vi "CRYUnits Conversion.vi"(7 "Axis to change units":enum16{"x", "y", "z"}(ring), 8 "New dB ref":dbl=1.0 format="%.1f", 9 "Custom unit in":string, 10 "New data (dB/Lin)":u16(ring)=1 items=["dB", "Lin"], 11 "Data in":T1={"Name"="", "Curve"=[], "X data"=1, "Y data"=1, "Z data"=1, "X axis"=0, "Y axis"=1, "Z axis"=1, "X unit"="Hz", "Y unit"="", "Z unit"="deg.", "X dB ref"=1.0, "Y dB ref"=1.0, "Z dB ref"=1.0, "single val"=FALSE, "protected"=FALSE, "display X"=TRUE, "display Y"=TRUE, "display Z"=TRUE, "Test Info"="", "Step No."=0, "Plot Settings"={"Color"=0, "Interpolation"=0, "Point Style"=0, "Line Style"=0, "Point Color"=0, "Line Width"=0, "Bar Plot Style"=0, "Fill To"=0}, "AutoProtect"=FALSE} {"Z data" items=["dB", "Lin"]; "X data" items=["dB", "Lin"]; "Y data" items=["dB", "Lin"]; "Z dB ref" format="%.1f"; "Z axis" items=["Log", "Lin"]; "X dB ref" format="%.1f"; "X axis" items=["Log", "Lin"]; "Y axis" items=["Log", "Lin"]; "Y dB ref" format="%.1f"; "Curve"."z" format="%.2f"; "Curve"."y" format="%.2f"; "Curve"."x" format="%.2f"}) -> (3 "Data with new units":T1={"Name"="", "Curve"=[], "X data"=1, "Y data"=1, "Z data"=1, "X axis"=0, "Y axis"=1, "Z axis"=1, "X unit"="Hz", "Y unit"="", "Z unit"="deg.", "X dB ref"=1.0, "Y dB ref"=1.0, "Z dB ref"=1.0, "single val"=FALSE, "protected"=FALSE, "display X"=TRUE, "display Y"=TRUE, "display Z"=TRUE, "Test Info"="", "Step No."=0, "Plot Settings"={"Color"=0, "Interpolation"=0, "Point Style"=0, "Line Style"=0, "Point Color"=0, "Line Width"=0, "Bar Plot Style"=0, "Fill To"=0}, "AutoProtect"=FALSE} {"Z data" items=["dB", "Lin"]; "X data" items=["dB", "Lin"]; "Y data" items=["dB", "Lin"]; "Z dB ref" format="%.1f"; "Z axis" items=["Log", "Lin"]; "X dB ref" format="%.1f"; "X axis" items=["Log", "Lin"]; "Y axis" items=["Log", "Lin"]; "Y dB ref" format="%.1f"; "Curve"."z" format="%.2f"; "Curve"."y" format="%.2f"; "Curve"."x" format="%.2f"})   [LabVIEW 2013]
uses:
  Typedef Control/CRYData Cluster.ctl
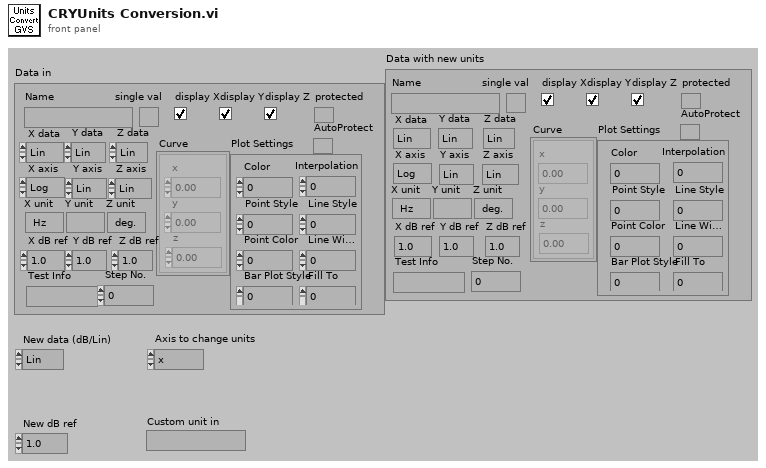
[diagram p1: front panel]
types:
  T1 = typedef "CRYData Cluster.ctl" = cluster{"Name":string, "Curve":cluster{"x":dbl, "y":dbl, "z":dbl}[], "X data":u16, "Y data":u16, "Z data":u16, "X axis":u16, "Y axis":u16, "Z axis":u16, "X unit":string, "Y unit":string, "Z unit":string, "X dB ref":dbl, "Y dB ref":dbl, "Z dB ref":dbl, "single val":bool, "protected":bool, "display X":bool, "display Y":bool, "display Z":bool, "Test Info":string, "Step No.":i32, "Plot Settings":cluster{"Color":u32, "Interpolation":u8, "Point Style":u8, "Line Style":u8, "Point Color":u32, "Line Width":u8, "Bar Plot Style":u8, "Fill To":i16}, "AutoProtect":bool}
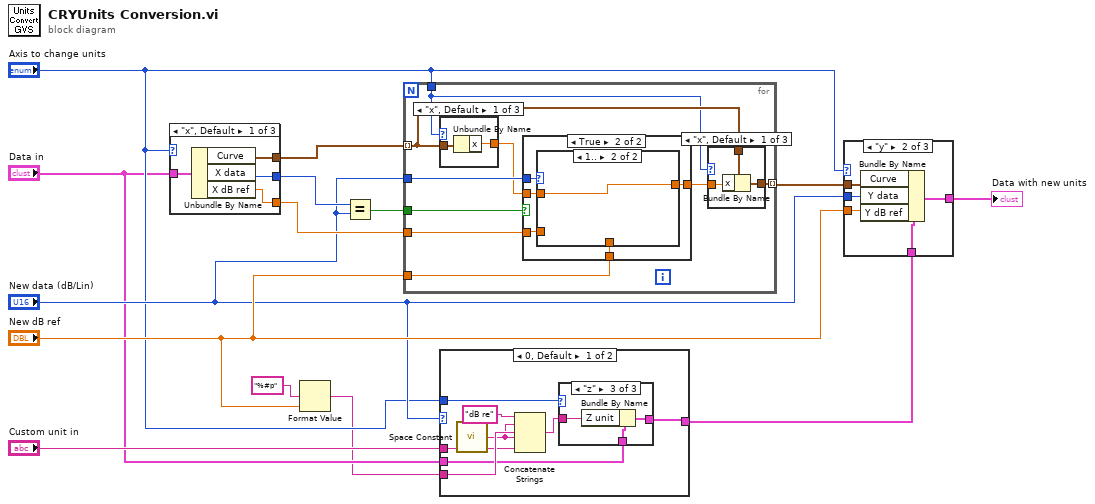
[diagram p0: block diagram]
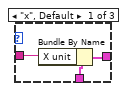
[diagram p2: hidden frame]
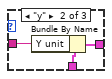
[diagram p3: hidden frame]
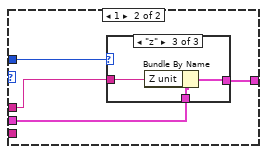
[diagram p4: hidden frame]
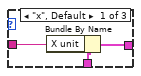
[diagram p5: hidden frame]
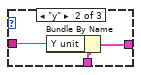
[diagram p6: hidden frame]
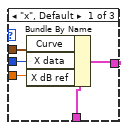
[diagram p7: hidden frame]
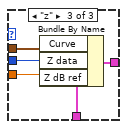
[diagram p8: hidden frame]
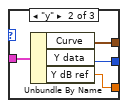
[diagram p9: hidden frame]
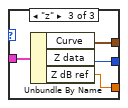
[diagram p10: hidden frame]
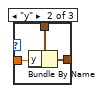
[diagram p11: hidden frame]
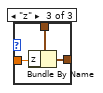
[diagram p12: hidden frame]
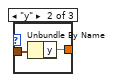
[diagram p13: hidden frame]
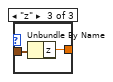
[diagram p14: hidden frame]
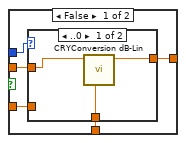
[diagram p15: hidden frame]
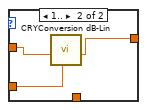
[diagram p16: hidden frame]
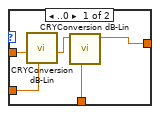
[diagram p17: hidden frame]
diagram:
  n1 = case shown="\"x\", Default" "Axis to change units" {
    tunnel: [w18 w22 w26] -> w12
    tunnel: [w17 w21 w25] -> w10
    tunnel: "Data in" -> [w16 w20 w24]
    tunnel: [w15 w19 w23] -> w11
    frame "x", Default {
      n2 = Unbundle By Name(w16) -> ("Curve"=w15:cluster{"x":dbl, "y":dbl, "z":dbl}[], "X data"=w17:u16, "X dB ref"=w18:dbl)
    }
    frame "y" {
      n3 = Unbundle By Name(w20) -> ("Curve"=w19:cluster{"x":dbl, "y":dbl, "z":dbl}[], "Y data"=w21:u16, "Y dB ref"=w22:dbl)
    }
    frame "z" {
      n4 = Unbundle By Name(w24) -> ("Curve"=w23:cluster{"x":dbl, "y":dbl, "z":dbl}[], "Z data"=w25:u16, "Z dB ref"=w26:dbl)
    }
  }
  n5 = Format Value(format string="%#p", value (0)="New dB ref") -> (output string=w2:string)  [unwired: 1 out]
  n6 = Equal?(x=w10, y="New data (dB/Lin)") -> (x = y?=w14:bool)
  n7 = for {
    tunnel: w14 -> [w35]
    tunnel: w11 -> [w32] mode=indexing
    tunnel: "New dB ref" -> [w29]
    tunnel: w12 -> [w34]
    tunnel: "New data (dB/Lin)" -> [w33]
    tunnel: [w30] -> w13 mode=indexing
    tunnel: "Axis to change units" -> [w27]
    n8 = case shown="\"x\", Default" w27 {
      tunnel: w32 -> [w46 w48 w50]
      tunnel: [w45 w47 w49] -> w28
      frame "x", Default {
        n9 = Unbundle By Name(w46) -> ("x"=w45:dbl)
      }
      frame "y" {
        n10 = Unbundle By Name(w48) -> ("y"=w47:dbl)
      }
      frame "z" {
        n11 = Unbundle By Name(w50) -> ("z"=w49:dbl)
      }
    }
    n12 = case shown="True" w35 {
      tunnel: [w55 w66] -> w31
      tunnel: w28 -> [w54 w65]
      tunnel: w29 -> [w53 w63]
      tunnel: w34 -> [w52 w62]
      tunnel: w33 -> [w51 w64]
      frame False {
        n13 = case shown="..0" w51 {
          tunnel: w53 -> [w58 _]
          tunnel: w54 -> [w56 w60]
          tunnel: [w57 w59] -> w55
          tunnel: w52 -> [_ w61]
          frame ..0 {
            n14 = call "CRYConversion dB-Lin.vi"("dB ref."=w58, "Lin In"=w56) -> ("Log Out"=w57:dbl)  [unwired: 4 in, 3 out]
          }
          frame 1.. {
            n15 = call "CRYConversion dB-Lin.vi"("dB ref."=w61, "Log In"=w60) -> ("Lin Out"=w59:dbl)  [unwired: 4 in, 3 out]
          }
        }
      }
      frame True {
        n16 = case shown="1.." w64 {
          tunnel: w65 -> [w71 w72]
          tunnel: [w69 w72] -> w66
          tunnel: w63 -> [w68 _]
          tunnel: w62 -> [w70 _]
          frame ..0 {
            n17 = call "CRYConversion dB-Lin.vi"("dB ref."=w70, "Log In"=w71) -> ("Lin Out"=w67:dbl)  [unwired: 4 in, 3 out]
            n18 = call "CRYConversion dB-Lin.vi"("dB ref."=w68, "Lin In"=w67) -> ("Log Out"=w69:dbl)  [unwired: 4 in, 3 out]
          }
          frame 1.. {
          }
        }
      }
    }
    n19 = case shown="\"x\", Default" w27 {
      tunnel: w32 -> [w38 w41 w44]
      tunnel: w31 -> [w37 w40 w43]
      tunnel: [w36 w39 w42] -> w30
      frame "x", Default {
        n20 = Bundle By Name(cluster=w38, "x"=w37) -> (w36:cluster{"x":dbl, "y":dbl, "z":dbl})
      }
      frame "y" {
        n21 = Bundle By Name(cluster=w41, "y"=w40) -> (w39:cluster{"x":dbl, "y":dbl, "z":dbl})
      }
      frame "z" {
        n22 = Bundle By Name(cluster=w44, "z"=w43) -> (w42:cluster{"x":dbl, "y":dbl, "z":dbl})
      }
    }
  }
  n23 = case shown="0, Default" "New data (dB/Lin)" {
    tunnel: "Custom unit in" -> [w75 w93]
    tunnel: [w79 w92] -> w1
    tunnel: w2 -> [w77 _]
    tunnel: "Data in" -> [w74 w91]
    tunnel: "Axis to change units" -> [w73 w90]
    frame 0, Default {
      n24 = call <vilib>:"Space Constant.vi"() -> ("String"=w76:string)
      n25 = Concatenate Strings("dB re" ("string"), w76, w77, w76, w75) -> (w80:string)
      n26 = case shown="\"z\"" w73 {
        tunnel: w80 -> [w83 w86 w89]
        tunnel: [w81 w85 w87] -> w79
        tunnel: w74 -> [w82 w84 w88]
        frame "x", Default {
          n27 = Bundle By Name(cluster=w82, "X unit"=w83) -> (w81:T1)
        }
        frame "y" {
          n28 = Bundle By Name(cluster=w84, "Y unit"=w86) -> (w85:T1)
        }
        frame "z" {
          n29 = Bundle By Name(cluster=w88, "Z unit"=w89) -> (w87:T1)
        }
      }
    }
    frame 1 {
      n30 = case shown="\"z\"" w90 {
        tunnel: w93 -> [w96 w99 w102]
        tunnel: [w94 w98 w100] -> w92
        tunnel: w91 -> [w95 w97 w101]
        frame "x", Default {
          n31 = Bundle By Name(cluster=w95, "X unit"=w96) -> (w94:T1)
        }
        frame "y" {
          n32 = Bundle By Name(cluster=w97, "Y unit"=w99) -> (w98:T1)
        }
        frame "z" {
          n33 = Bundle By Name(cluster=w101, "Z unit"=w102) -> (w100:T1)
        }
      }
    }
  }
  n34 = case shown="\"y\"" "Axis to change units" {
    tunnel: w13 -> [w107 w112 w117]
    tunnel: w1 -> [w106 w111 w116]
    tunnel: "New data (dB/Lin)" -> [w105 w110 w115]
    tunnel: "New dB ref" -> [w104 w109 w114]
    tunnel: [w103 w108 w113] -> w9
    frame "x", Default {
      n35 = Bundle By Name(cluster=w106, "Curve"=w107, "X data"=w105, "X dB ref"=w104) -> (w103:T1)
    }
    frame "y" {
      n36 = Bundle By Name(cluster=w111, "Curve"=w112, "Y data"=w110, "Y dB ref"=w109) -> (w108:T1)
    }
    frame "z" {
      n37 = Bundle By Name(cluster=w116, "Curve"=w117, "Z data"=w115, "Z dB ref"=w114) -> (w113:T1)
    }
  }
  "Data with new units" <- w9
